vi "LV86_GetImageSubset.vi"(2 "ROI":T1, 3 "Image In":T2 {"Dialogs" format="%.0b"}) -> (1 "Image out":T2 {"Dialogs" format="%.0b"})   [LabVIEW 2024]
doc: "This VI extracts a subImage from the original image"
uses:
  <userlib>/ImageProcessing/QTLIB_2595_LV86/QT_Image.ctl
panel:
  # "This VI extracts a subImage from the original image"
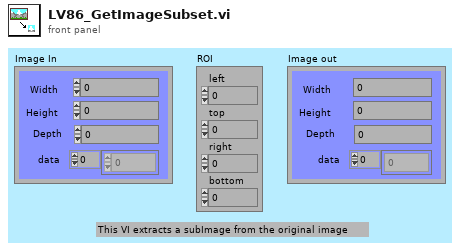
[diagram p1: front panel]
types:
  T1 = cluster{"left":i32, "top":i32, "right":i32, "bottom":i32}
  T2 = typedef "QT_Image.ctl" = cluster{"Width":i32, "Height":i32, "Depth":i32, "data":u8[], "Compressed data":u8[], "Color table":u32[], "Duration":i32, "Options":i32, "Timestamp":i32, "ID":i32, "Reserved":i32, "Dialogs":u32}
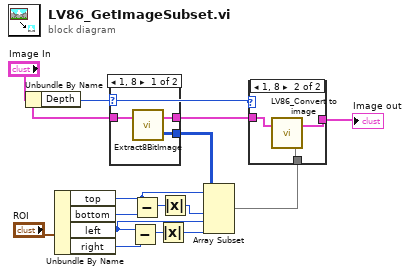
[diagram p0: block diagram]
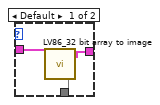
[diagram p2: hidden frame]
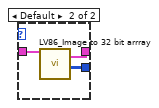
[diagram p3: hidden frame]
diagram:
  n1 = Unbundle By Name("Image In") -> ("Depth"=w1:i32)
  n2 = Unbundle By Name("ROI") -> ("top"=w10:i32, "bottom"=w11:i32, "left"=w4:i32, "right"=w7:i32)
  n3 = case shown="1, 8" w1 {
    tunnel: "Image In" -> [w17 w21]
    tunnel: [w16 w20] -> w12
    tunnel: [w18 w19] -> w6
    frame 1, 8 {
      n4 = call <userlib>:"Extract8BitImage.vi"("Image in"=w17) -> ("Intensity Graph"=w18:u8[][], "Image out"=w16:T2)  [unwired: 1 in]
    }
    frame Default {
      n5 = call <userlib>:"LV86_Image to 32 bit arrray.vi"("Image In"=w21) -> ("Intensity Graph"=w19:u32[][], "Image out"=w20:T2)  [unwired: 1 in]
    }
  }
  n6 = Subtract(x=w4, y=w7) -> (x-y=w8:i32)
  n7 = Subtract(x=w10, y=w11) -> (x-y=w9:i32)
  n8 = Absolute Value(x=w8) -> (abs(x)=w2:i32)
  n9 = Absolute Value(x=w9) -> (abs(x)=w3:i32)
  n10 = Array Subset(array=w6, index (row)=w10, length (row)=w3, index (col)=w4, length (col)=w2) -> (w5:u32[][])
  n11 = case shown="1, 8" w1 {
    tunnel: w12 -> [w24 w27]
    tunnel: [w23 w26] -> w15
    tunnel: w5 -> [w22 w25]
    frame Default {
      n12 = call <userlib>:"LV86_32 bit array to image.vi"("Intensity Graph"=w22, "Image In"=w24) -> ("Image Out"=w23:T2)  [unwired: 1 in]
    }
    frame 1, 8 {
      n13 = call <userlib>:"LV86_Convert to image.vi"("Intensity Graph"=w25, "Image In"=w27) -> ("Image Out"=w26:T2)  [unwired: 1 in]
    }
  }
  "Image out" <- w15
